vi "Linsenberechnung.vi"() -> ()   [LabVIEW 2013]
panel:
  out "I_var_2":dbl
  out "I_var_1":dbl
  out "f_var_2":dbl
  out "f_var_1":dbl
  out "M":dbl
  in  "stop":bool
  out "f_2":dbl
  out "f_1":dbl
  in  "Vergrößerung":dbl(slide) scale=0.0..10.0
  out "M_min":dbl=0.6250000000000001
  out "M_max":dbl=0.8
  out "f_1_max_real":dbl=35.55555555555556
  out "f_2_max_real":dbl=49.230769230769226
  in  "Eigener Abstand e":dbl=80.0 format="%#_13g"
  out "Vorgeschlagener Abstand Linsen e":dbl=91.17826617826617
  in  "f_offset 2":dbl=50.0
  out "f_2_min":dbl=44.44444444444444
  out "f_2_max":dbl=71.42857142857143
  out "f_1_min":dbl=30.76923076923077
  out "f_1_max":dbl=35.714285714285715
  in  "f_min":dbl=80.0
  in  "f_offset 1":dbl=100.0
  in  "f_max":dbl=200.0
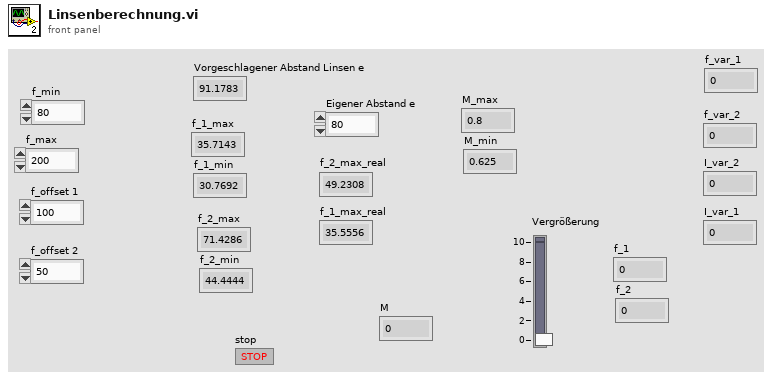
[diagram p1: front panel]
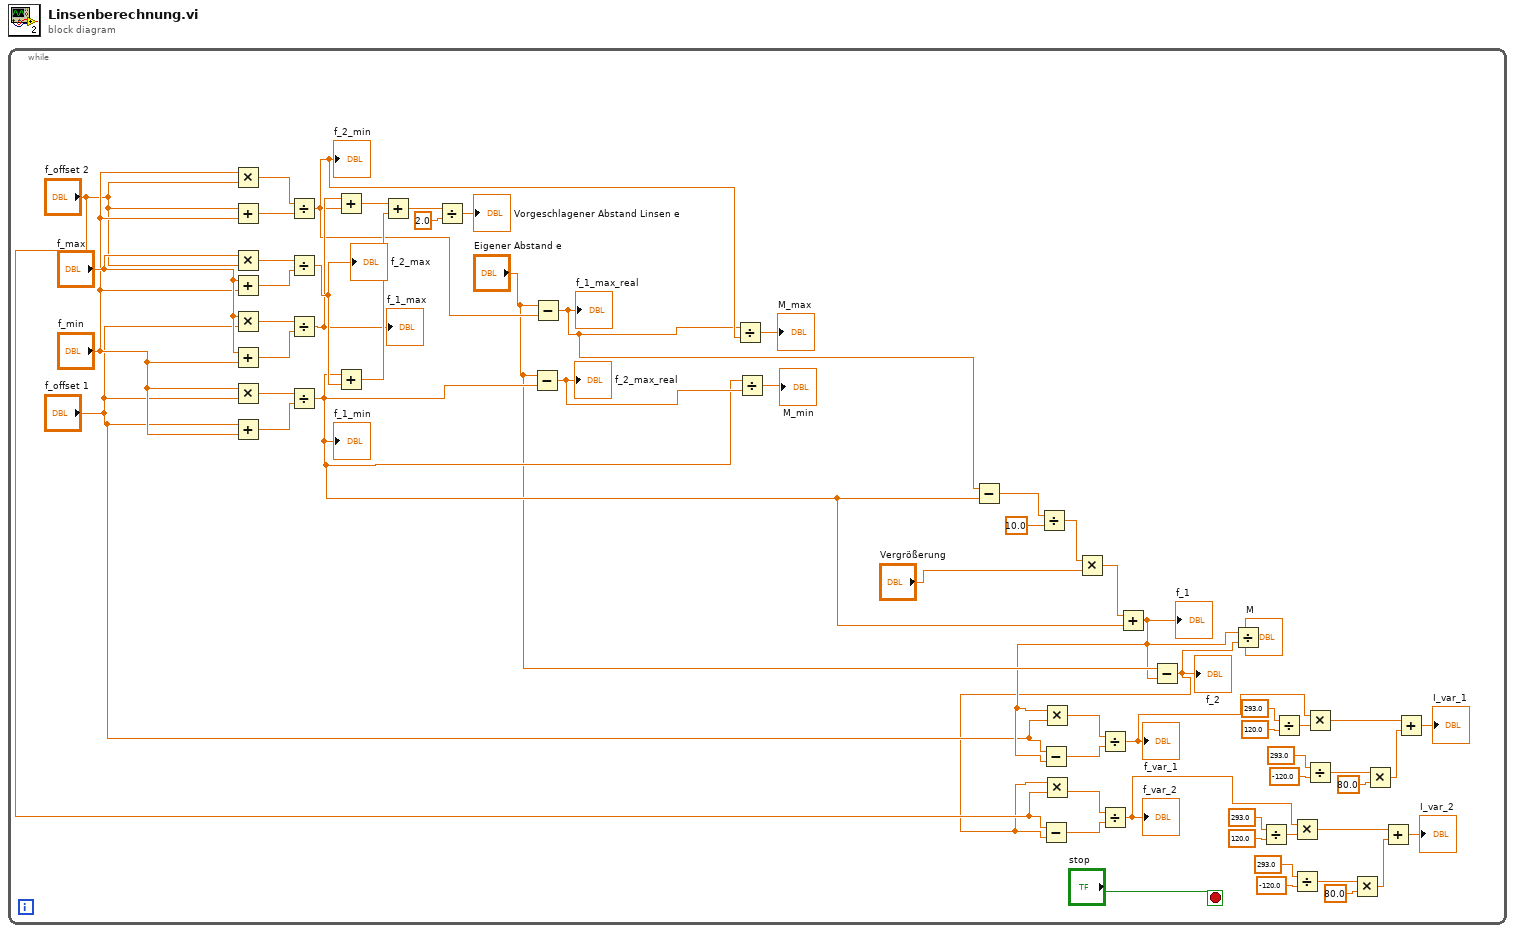
[diagram p0: block diagram]
diagram:
  n1 = while {
    stop <- "stop" stop-if-true
    n2 = Multiply(x="f_min", y="f_offset 2") -> (x*y=w56:dbl)
    n3 = Add(x="f_offset 2", y="f_min") -> (x+y=w57:dbl)
    n4 = Multiply(x="f_max", y="f_offset 2") -> (x*y=w54:dbl)
    n5 = Add(x="f_max", y="f_min") -> (x+y=w55:dbl)
    n6 = Multiply(x="f_max", y="f_offset 1") -> (x*y=w58:dbl)
    n7 = Add(x="f_max", y="f_min") -> (x+y=w59:dbl)
    n8 = Multiply(x="f_min", y="f_offset 1") -> (x*y=w60:dbl)
    n9 = Add(x="f_offset 1", y="f_min") -> (x+y=w61:dbl)
    n10 = Divide(x=w56, y=w57) -> (x/y=w43:dbl)
    "f_2_min" <- w43
    n11 = Divide(x=w54, y=w55) -> (x/y=w46:dbl)
    "f_2_max" <- w46
    n12 = Divide(x=w58, y=w59) -> (x/y=w45:dbl)
    "f_1_max" <- w45
    n13 = Divide(x=w60, y=w61) -> (x/y=w34:dbl)
    "f_1_min" <- w34
    n14 = Add(x=w45, y=w43) -> (x+y=w50:dbl)
    n15 = Add(x=w34, y=w46) -> (x+y=w49:dbl)
    n16 = Add(x=w50, y=w49) -> (x+y=w48:dbl)
    n17 = Divide(x=w48, y=2.0) -> (x/y=→"Vorgeschlagener Abstand Linsen e":dbl)
    n18 = Subtract(x="Eigener Abstand e", y=w34) -> (x-y=w44:dbl)
    "f_2_max_real" <- w44
    n19 = Subtract(x="Eigener Abstand e", y=w43) -> (x-y=w40:dbl)
    "f_1_max_real" <- w40
    n20 = Divide(x=w40, y=w43) -> (x/y=→"M_max":dbl)
    n21 = Divide(x=w34, y=w44) -> (x/y=→"M_min":dbl)
    n22 = Subtract(x=w40, y=w34) -> (x-y=w39:dbl)
    n23 = Divide(x=w39, y=10.0) -> (x/y=w37:dbl)
    n24 = Multiply(x=w37, y="Vergrößerung") -> (x*y=w35:dbl)
    n25 = Add(x=w35, y=w34) -> (x+y=w28:dbl)
    "f_1" <- w28
    n26 = Subtract(x="f_offset 1", y=w28) -> (x-y=w29:dbl)
    n27 = Multiply(x=w28, y="f_offset 1") -> (x*y=w30:dbl)
    n28 = Divide(x=w30, y=w29) -> (x/y=w13:dbl)
    "f_var_1" <- w13
    n29 = Subtract(x="Eigener Abstand e", y=w28) -> (x-y=w23:dbl)
    "f_2" <- w23
    n30 = Subtract(x="f_offset 2", y=w23) -> (x-y=w25:dbl)
    n31 = Multiply(x=w23, y="f_offset 2") -> (x*y=w26:dbl)
    n32 = Divide(x=w26, y=w25) -> (x/y=w1:dbl)
    "f_var_2" <- w1
    n33 = Divide(x=w28, y=w23) -> (x/y=→"M":dbl)
    n34 = Divide(x=293.0, y=120.0) -> (x/y=w4:dbl)
    n35 = Divide(x=293.0, y=120.0) -> (x/y=w15:dbl)
    n36 = Multiply(x=w1, y=w4) -> (x*y=w3:dbl)
    n37 = Divide(x=293.0, y=-120.0) -> (x/y=w6:dbl)
    n38 = Multiply(x=w13, y=w15) -> (x*y=w14:dbl)
    n39 = Divide(x=293.0, y=-120.0) -> (x/y=w17:dbl)
    n40 = Multiply(x=w6, y=80.0) -> (x*y=w7:dbl)
    n41 = Multiply(x=w17, y=80.0) -> (x*y=w18:dbl)
    n42 = Add(x=w3, y=w7) -> (x+y=→"I_var_2":dbl)
    n43 = Add(x=w14, y=w18) -> (x+y=→"I_var_1":dbl)
  }
